vi "PH_VacuumControl.evt Set Unit.vi"(0 "i ref in":refnum<vi>, 1 "Instance":string="N/A", 2 "Unit":i32(ring)=1 items=["mBar", "Pascal", "Torr"], 5 "error in (no error)":errorcluster) -> (14 "i ref out":refnum<vi>, 19 "error out":errorcluster)   [LabVIEW 2014, in "PH_VacuumControl.lvlib"]
doc: "This VI sends a command to play a tone"
uses:
  PH_VacuumControl.lvlib
  CS_Core/CSSystem/CoreLib/CoreLib.int 2 byte array.vi
  CS_Core/CSSystem/CoreLib/CoreLib.lvlib
  CS_Core/BaseProcess/BaseProcess.lvlib
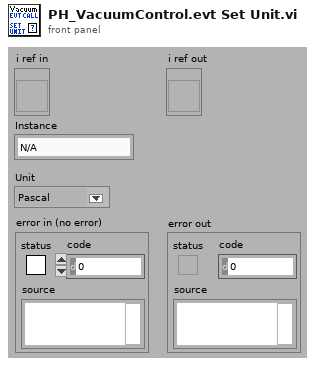
[diagram p1: front panel]
types:
  T1 = typedef "CoreDefs.rawDataType.ctl" = i8[]
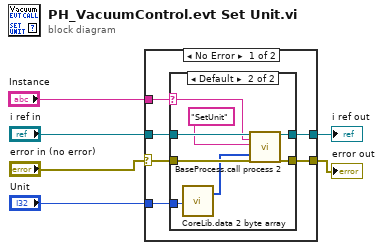
[diagram p0: block diagram]
diagram:
  n1 = case shown="No Error" "error in (no error)" {
    selector: "error in (no error)" -> [w7 w23]
    tunnel: [w12 w24] -> w6
    tunnel: [w11 w23] -> w5
    tunnel: "i ref in" -> [w10 w24]
    tunnel: "Instance" -> [w9 _]
    tunnel: "Unit" -> [w8 _]
    frame No Error {
      n2 = case shown="Default" w9 {
        selector: w9 -> [_ w18]
        tunnel: [w14 w22] -> w12
        tunnel: [w13 w21] -> w11
        tunnel: w10 -> [w14 w20]
        tunnel: w7 -> [w13 w19]
        tunnel: w8 -> [_ w16]
        frame "N/A" {
        }
        frame Default {
          n3 = call-poly "CoreLib.data 2 byte array.vi"("i32"=w16) -> ("byteArray out"=w15:T1)  [unwired: 18 in]
          n4 = call "BaseProcess.call process 2.vi"("i ref in"=w20, "Object"=w18, "Selector"="SetUnit", "Data"=w15, "error in (no error)"=w19) -> ("i ref out"=w22:refnum<vi>, "error out"=w21:errorcluster)  [unwired: 13 in]
        }
      }
    }
    frame Error {
    }
  }
  "error out" <- w5
  "i ref out" <- w6
